vi "Command to write.vi"(11 "Set Points":dbl[](array[numeric])=[1.0]) -> (2 "Unit ID":i32, 3 "Command to write":string)   [LabVIEW 2015]
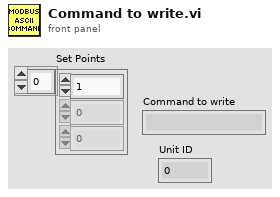
[diagram p1: front panel]
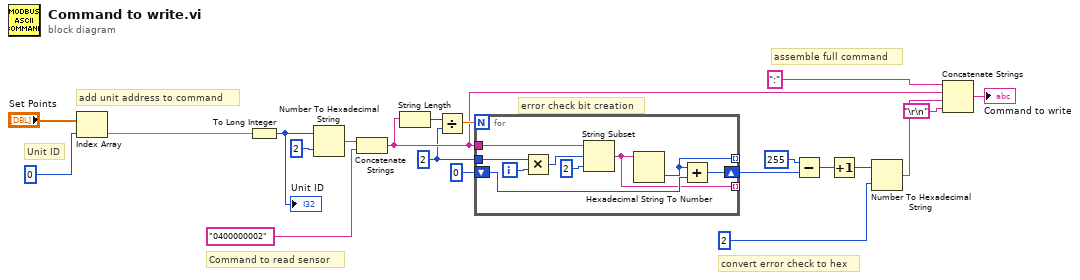
[diagram p0: block diagram]
diagram:
  w2 = 2 ("y")
  # "add unit address to command"
  # "assemble full command"
  # "convert error check to hex"
  # "error check bit creation"
  # "Command to read sensor"
  # "Unit ID"
  n1 = Index Array(array="Set Points", index=0) -> (element=w1:dbl)
  n2 = To Long Integer(number=w1) -> (32bit integer=w8:i32)
  "Unit ID" <- w8
  n3 = Number To Hexadecimal String(1:i16 2 ("width (-)"), 2:w8) -> (0:w11:string)
  n4 = Concatenate Strings(w11, "0400000002" ("command")) -> (w3:string)
  n5 = String Length(string=w3) -> (length=w5:i32)
  n6 = Divide(x=w5, y=w2) -> (x/y=w6:dbl)
  n7 = for {
    N: w6 -> [_]
    tunnel: w3 -> [w27]
    shift-right: [w29] -> w19
    shift-left: u8 0 -> [w30]
    tunnel: [w28] -> _ mode=indexing
    tunnel: w2 -> [w23]
    tunnel: [w22] -> _ mode=indexing
    i -> [w26]
    n8 = Multiply(x=w23, y=w26) -> (x*y=w24:i32)
    n9 = String Subset(string=w27, offset (0)=w24, length (rest)=2 ("length (rest)")) -> (substring=w22:string)
    n10 = Hexadecimal String To Number(string=w22) -> (number=w28:u32)  [unwired: 2 in, 1 out]
    n11 = Add(x=w28, y=w30) -> (x+y=w29:u32)
  }
  n12 = Subtract(x=255, y=w19) -> (x-y=w16:u32)
  n13 = Increment(x=w16) -> (x+1=w17:u32)
  n14 = Number To Hexadecimal String(1:i16 2 ("width (-)"), 2:w17) -> (0:w4:string)
  n15 = Concatenate Strings(":" ("string"), w3, w4, "\r\n") -> (→"Command to write":string)
